vi "RotationApplication V4.vi"() -> ()   [LabVIEW 2012]
uses:
  <instrlib>/ZaberTSeries/Public/Utility/Request.ctl
  <instrlib>/ZaberTSeries/Public/Utility/Response.ctl
  Stage Global.vi
  <instrlib>/ZaberTSeries/ZaberTSeries.lvlib
panel:
  out "Scanning?":bool
  out "Current Angle (deg)":dbl=45.0
  out "Stage Position (mm)":dbl=75.00015258789062
  in  "Time Step (ms)":dbl
  in  "Rotation f(x) (mm -> deg)":string="2.7355608145532777*x*x*x*x*x*x - 1187.125773554726*x*x*x*x*x + 214643.38075449364*x*x*x*x - 20697537.088212848*x*x*x + 1122597496.9922702*x*x - 32472066742.439888*x + 391350879609.55573"
  in  "Finish Rotation f(x)":bool
  in  "Scan":bool
  in  "stop":bool
  in  "Go Home":bool
  in  "Set Home Offset":dbl=89.0
  in  "?":T1(tab)
  in  "Optimize":bool
  in  "Angle?":bool
  out "Current Angle (deg)":dbl=38.0090625
  in  "Move Rel?":bool
  in  "Move Abs?":bool
  in  "Move Rel (deg)":dbl=-1.0 step=0.1
  in  "Move Abs (deg)":dbl=19.0
  in  "Send":bool
  out "Command?":bool
  in  "REQUEST:":T2={"Device Number"=1, "Command"=23, "Data"=-10000, "Response Count"=1} {"Command" items=["Echo"=55, "Home"=1, "Move Absolute"=20, "Move Relative"=21, "Move at Constant Speed"=22, "Renumber"=2, "Restore Settings"=36, "Stop"=23]}
  out "Response Data:":T3 {"Command" items=["Constant Speed Tracking"=8, "Echo"=55, "Error"=255, "Home"=1, "Limit Active"=9, "Manual Move Tracking"=10, "Move Absolute"=20, "Move at Constant Speed"=22, "Move Relative"=21, "Renumber"=2, "Restore Settings"=36, "Stop"=23]}
  in  "Command":bool
  in  "DONE":bool=TRUE
  in  "Simulation":bool
  out "Simulate?":bool
  in  "Finish Stage":bool
  in  "Start/pause":bool
  in  "Start/Pause Stage":bool
  out "Current Position (mm)":dbl
  in  "Finish Rotation":bool
  out "Current Angle":dbl
  in  "Initial Position (mm)":dbl
  in  "Final Position (mm)":dbl
  in  "Number of Steps":u32
  in  "Speed (um/s)":dbl
  in  "Final Angle (deg)":dbl=45.0
  in  "Number of Rotations":u32=4500
  in  "Polynomial Degree":dbl=1.0
  in  "VISA reference name:":refnum<visa-resource-name>="COM4"
  # "==>"
  # "Device"
  # "Command (Binary)"
  # "Data"
  # "==>"
  # "Data"
  # "==>"
  # "Rotation Mount Settings:"
  # "Simulated Delay Stage Settings:"
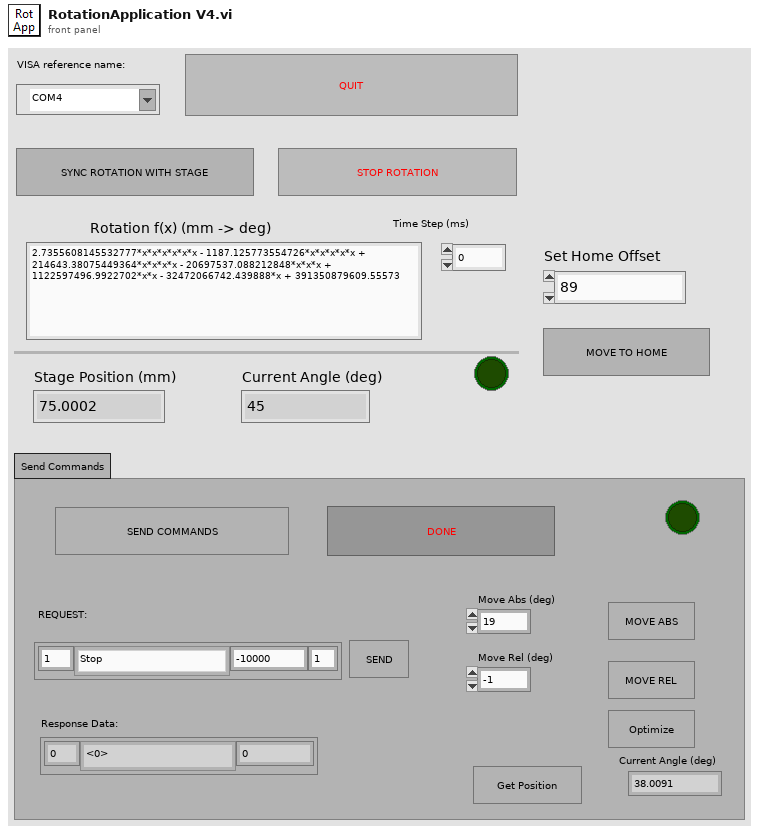
[diagram p1: front panel]
types:
  T1 = enum32{"Send Commands", "Simulated f(x)  ", "Adjust Simulation Settings"}
  T2 = typedef "ZaberTSeries.lvlib/Request.ctl" = cluster{"Device Number":u8, "Command":u8, "Data":i32, "Response Count":i32}
  T3 = typedef "ZaberTSeries.lvlib/Response.ctl" = cluster{"Device Number":u8, "Command":u8, "Data":i32}
  T4 = enum8{"Enabled", "Disabled", "Disabled and Grayed Out"}
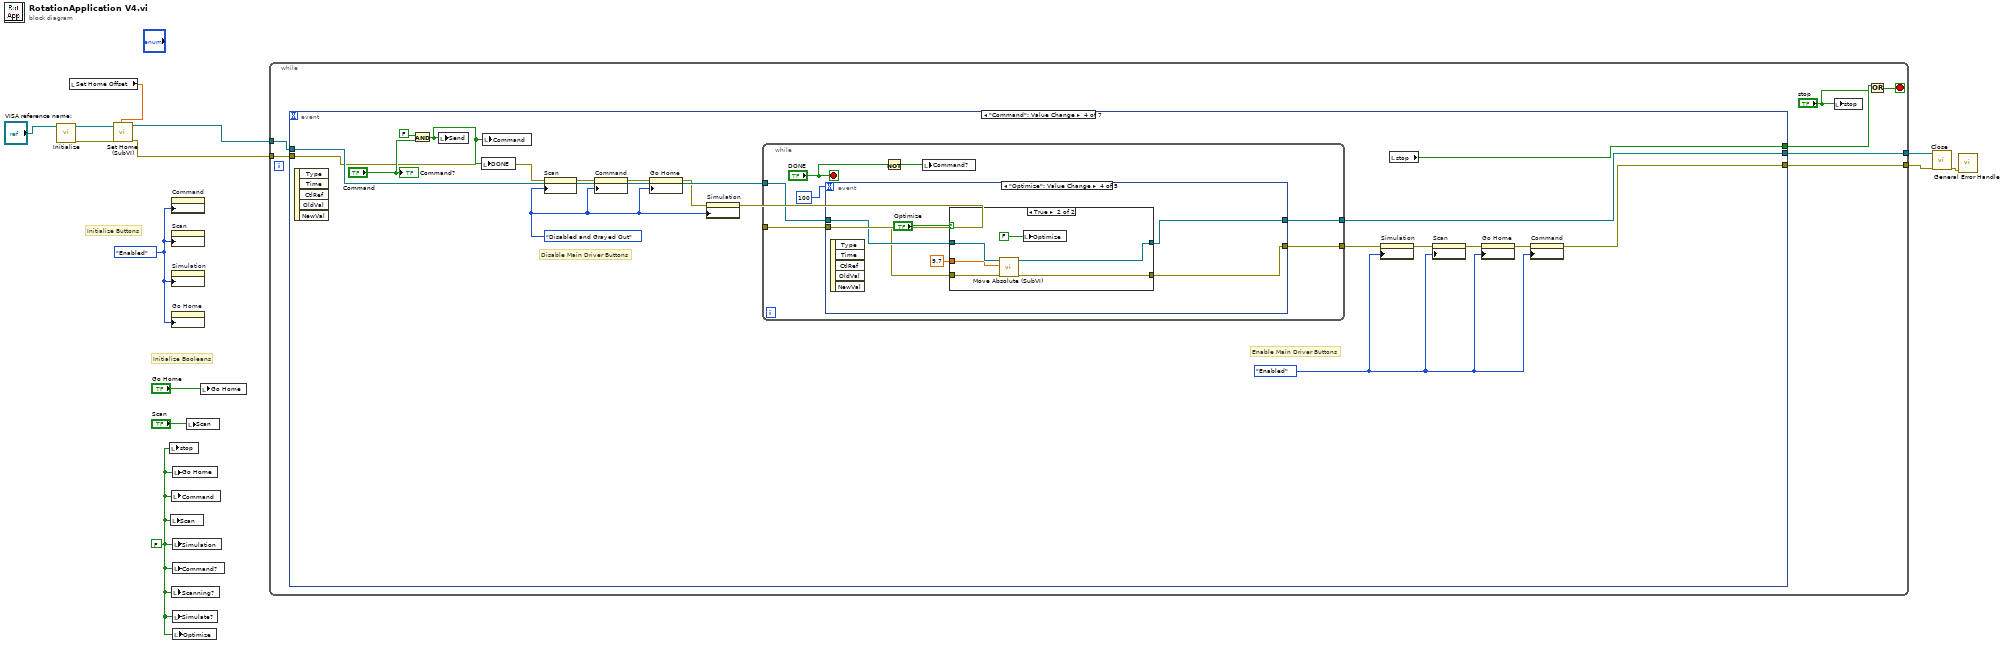
[diagram p0: block diagram]
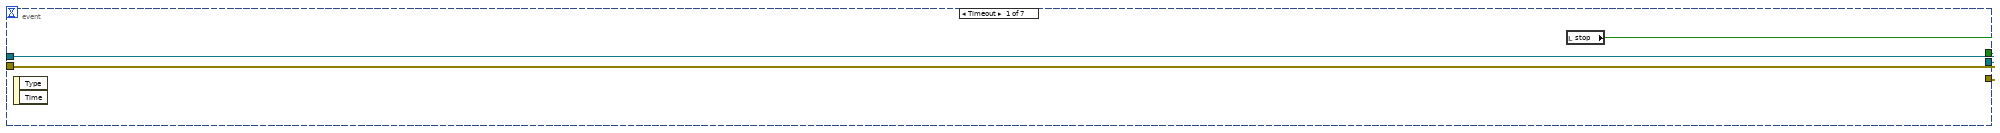
[diagram p2: hidden frame]
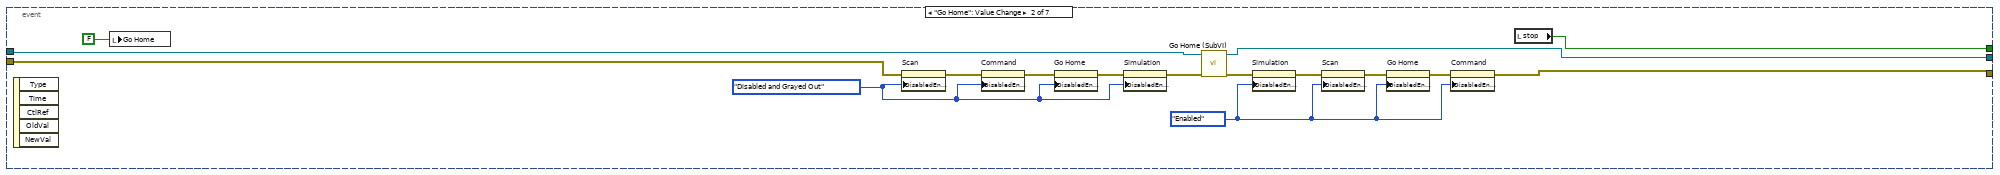
[diagram p3: hidden frame]
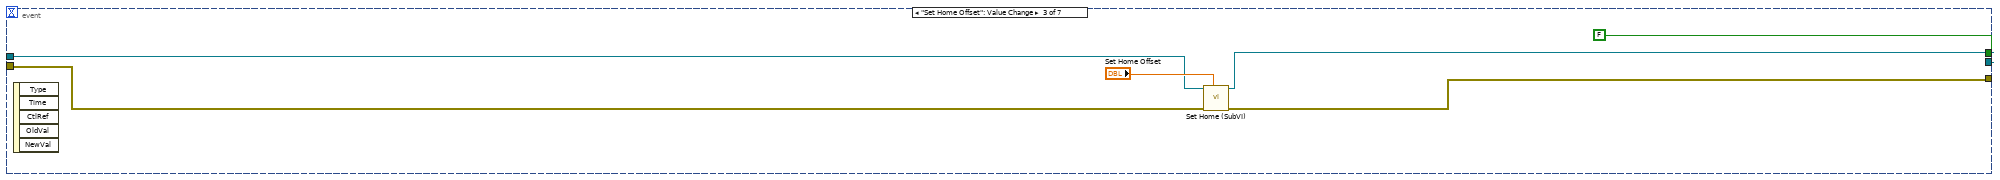
[diagram p4: hidden frame]
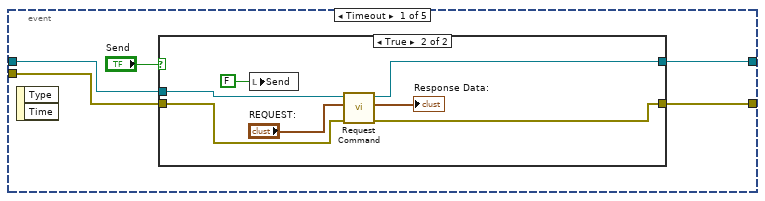
[diagram p5: hidden frame]
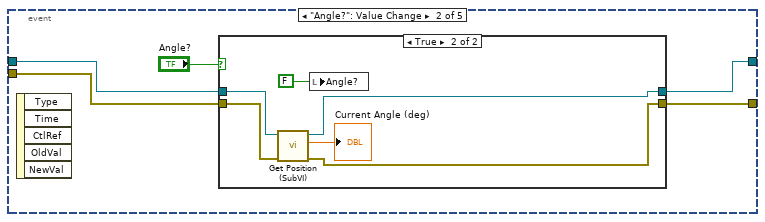
[diagram p7: hidden frame]
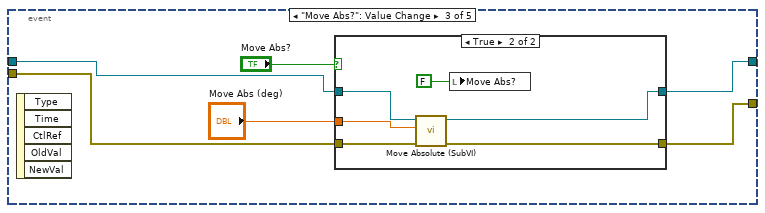
[diagram p9: hidden frame]
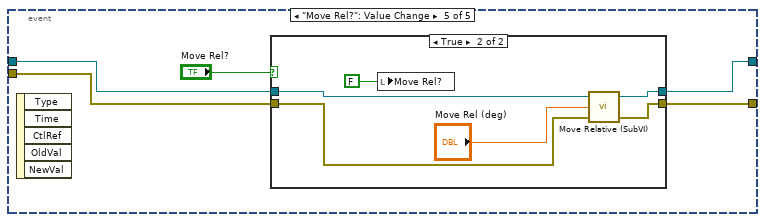
[diagram p12: hidden frame]
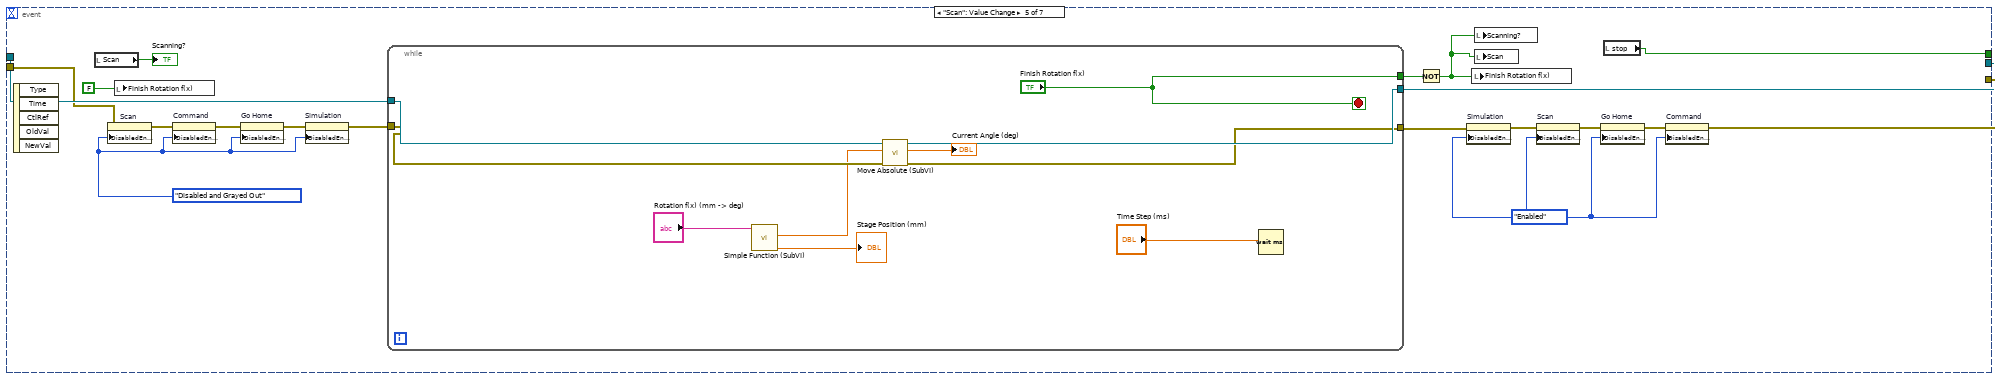
[diagram p14: hidden frame]
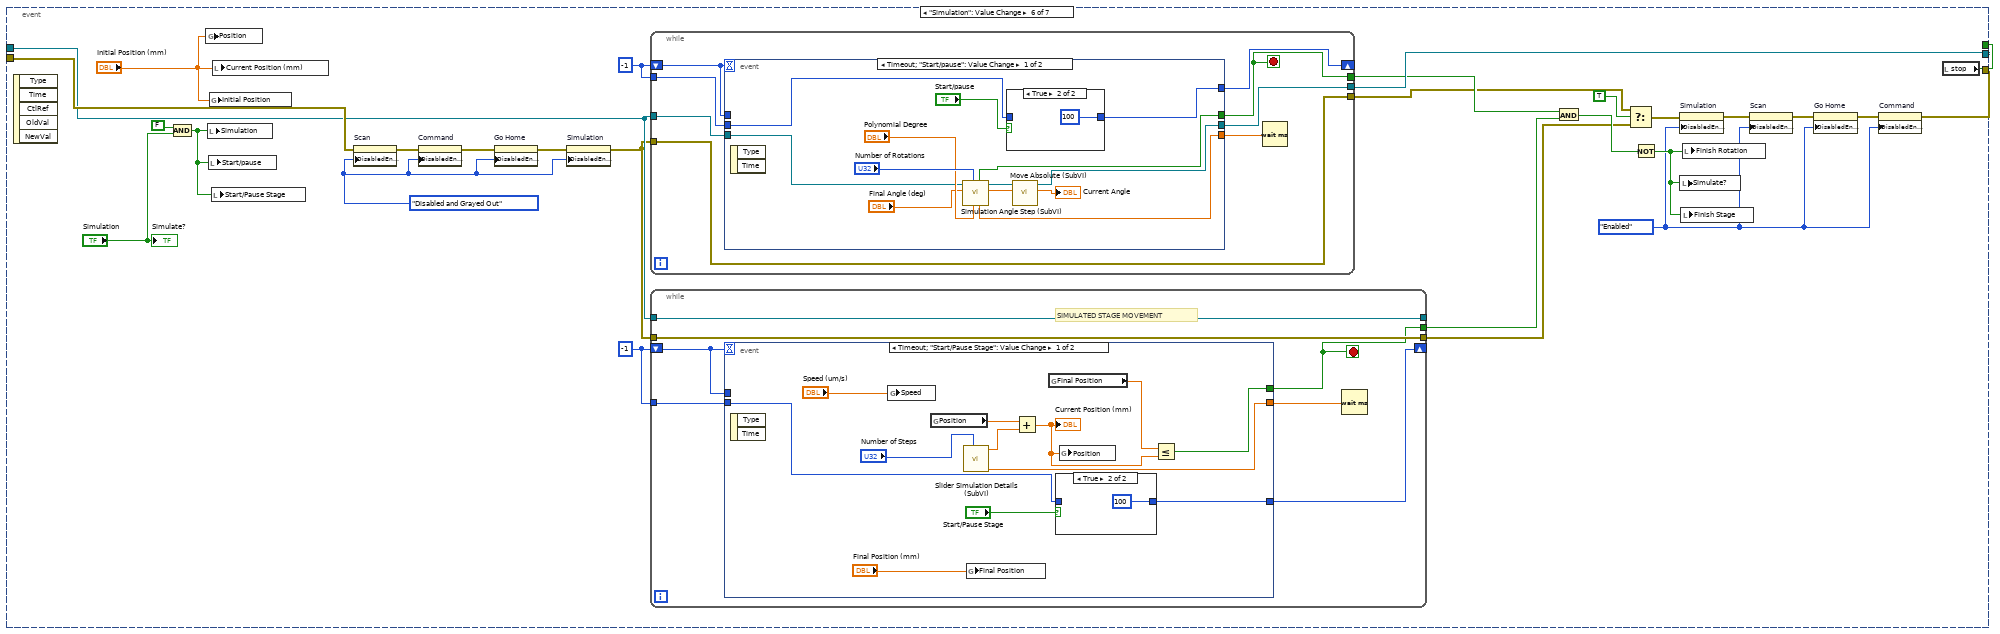
[diagram p15: hidden frame]
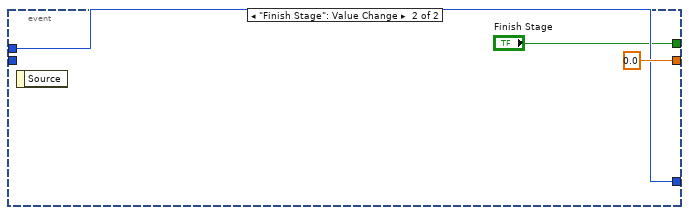
[diagram p17: hidden frame]
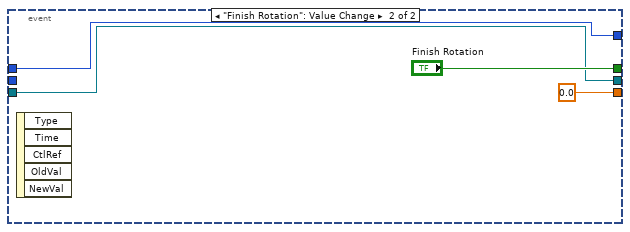
[diagram p19: hidden frame]
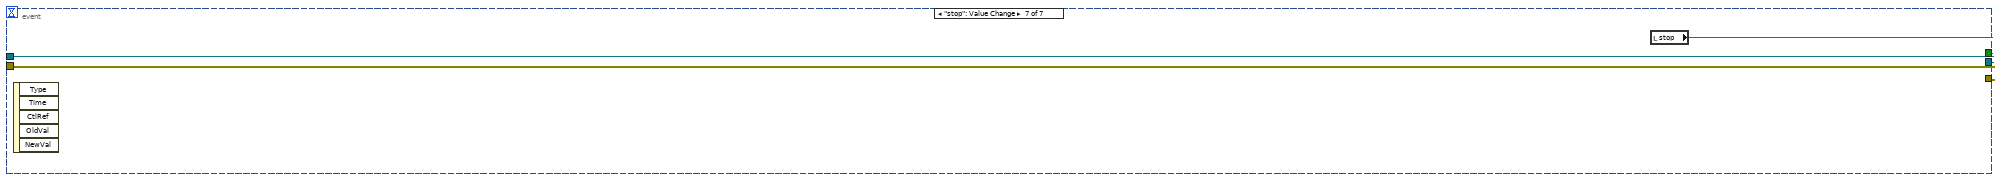
[diagram p20: hidden frame]
diagram:
  w9 = T4."Enabled" ("Disabled")
  w1 = FALSE ("y")
  # "Initialize Buttons"
  # "Initialize Booleans"
  n1 = call <instrlib>:"Initialize.vi"("VISA resource name"="VISA reference name:") -> ("error out"=w4:errorcluster, "VISA resource name out"=w6:refnum<visa-resource-name>)  [unwired: 8 in, 1 out]
  n2 = local read "Set Home Offset"() -> (w2:dbl)
  n3 = call "Set Home (SubVI).vi"("Home Offset (deg)"=w2, "error in (no error)"=w4, "VISA Refnum in"=w6) -> ("error out"=w3:errorcluster, "VISA Refnum out"=w5:refnum<visa-resource-name>)  [unwired: 7 in]
  n4 = local write "stop"(w1) -> ()
  n5 = local write "Scan"(w1) -> ()
  n6 = property on="Command" class="Bool (strict)"("DisabledEnum"=w9) -> ()  [unwired: 2 in, 2 out]
  n7 = property on="Scan" class="Bool (strict)"("DisabledEnum"=w9) -> ()  [unwired: 2 in, 2 out]
  n8 = property on="Simulation" class="Bool (strict)"("DisabledEnum"=w9) -> ()  [unwired: 2 in, 2 out]
  n9 = property on="Go Home" class="Bool (strict)"("DisabledEnum"=w9) -> ()  [unwired: 2 in, 2 out]
  n10 = local write "Command"(w1) -> ()
  n11 = local write "Scanning?"(w1) -> ()
  n12 = local write "Go Home"(w1) -> ()
  n13 = local write "Simulation"(w1) -> ()
  n14 = local write "Command?"(w1) -> ()
  n15 = local write "Simulate?"(w1) -> ()
  n16 = local write "Optimize"(w1) -> ()
  n17 = local write "Scan"("Scan") -> ()
  n18 = local write "Go Home"("Go Home") -> ()
  n19 = while {
    tunnel: w5 -> [w15]
    tunnel: w3 -> [w14]
    tunnel: [w20] -> w11
    tunnel: [w19] -> w13
    stop <- w18 stop-if-true
    n20 = event shown="[3] \"Command\": Value Change" {
      selector: _ -> [_ _ _ _ _ _ _]
      dyn-events: _ -> [_ _ _ _ _ _ _]
      timeout: _ -> [_ _ _ _ _ _ _]
      tunnel: w15 -> [w23 w34 w44 w63 w156 w183 w248]
      tunnel: w14 -> [w22 w25 w43 w47 w153 w192 w247]
      tunnel: [w23 w28 w42 w55 w155 w190 w248] -> w19
      tunnel: [w22 w29 w41 w51 w150 w187 w247] -> w20
      tunnel: [w21 w39 FALSE ("stop") w62 w157 w195 w249] -> w17
      event Timeout {
        n21 = event-data() -> ()  [unwired: 1 in, 2 out]
        n22 = local read "stop"() -> (w21:bool)
      }
      event "Go Home": Value Change {
        w26 = T4."Enabled" ("Disabled")
        w27 = T4."Disabled and Grayed Out" ("Disabled")
        n23 = event-data() -> ()  [unwired: 1 in, 5 out]
        n24 = local write "Go Home"(FALSE ("Go Home")) -> ()
        n25 = property on="Scan" class="Bool (strict)"(error in=w25, "DisabledEnum"=w27) -> (error out=w37:errorcluster)  [unwired: 1 in, 1 out]
        n26 = property on="Command" class="Bool (strict)"(error in=w37, "DisabledEnum"=w27) -> (error out=w36:errorcluster)  [unwired: 1 in, 1 out]
        n27 = property on="Go Home" class="Bool (strict)"(error in=w36, "DisabledEnum"=w27) -> (error out=w35:errorcluster)  [unwired: 1 in, 1 out]
        n28 = property on="Simulation" class="Bool (strict)"(error in=w35, "DisabledEnum"=w27) -> (error out=w33:errorcluster)  [unwired: 1 in, 1 out]
        n29 = call "Go Home (SubVI).vi"("error in (no error)"=w33, "VISA Refnum in"=w34) -> ("error out"=w24:errorcluster, "VISA Refnum out"=w28:refnum<visa-resource-name>)  [unwired: 8 in]
        n30 = property on="Simulation" class="Bool (strict)"(error in=w24, "DisabledEnum"=w26) -> (error out=w30:errorcluster)  [unwired: 1 in, 1 out]
        n31 = property on="Scan" class="Bool (strict)"(error in=w30, "DisabledEnum"=w26) -> (error out=w32:errorcluster)  [unwired: 1 in, 1 out]
        n32 = property on="Go Home" class="Bool (strict)"(error in=w32, "DisabledEnum"=w26) -> (error out=w31:errorcluster)  [unwired: 1 in, 1 out]
        n33 = property on="Command" class="Bool (strict)"(error in=w31, "DisabledEnum"=w26) -> (error out=w29:errorcluster)  [unwired: 1 in, 1 out]
        n34 = local read "stop"() -> (w39:bool)
      }
      event "Set Home Offset": Value Change {
        n35 = event-data() -> ()  [unwired: 1 in, 5 out]
        n36 = call "Set Home (SubVI).vi"("Home Offset (deg)"="Set Home Offset", "error in (no error)"=w43, "VISA Refnum in"=w44) -> ("error out"=w41:errorcluster, "VISA Refnum out"=w42:refnum<visa-resource-name>)  [unwired: 7 in]
      }
      event "Command": Value Change {
        w49 = T4."Enabled" ("Disabled")
        w50 = T4."Disabled and Grayed Out" ("Disabled")
        # "Enable Main Driver Buttons"
        # "Disable Main Driver Buttons"
        n37 = event-data() -> ()  [unwired: 1 in, 5 out]
        n38 = And(x=FALSE ("Command"), y="Command") -> (x .and. y?=w48:bool)
        n39 = local write "Send"(w48) -> ()
        n40 = local write "DONE"(w48) -> ()
        n41 = local write "Command"(w48) -> ()
        n42 = property on="Scan" class="Bool (strict)"(error in=w47, "DisabledEnum"=w50) -> (error out=w57:errorcluster)  [unwired: 1 in, 1 out]
        n43 = property on="Command" class="Bool (strict)"(error in=w57, "DisabledEnum"=w50) -> (error out=w58:errorcluster)  [unwired: 1 in, 1 out]
        n44 = property on="Go Home" class="Bool (strict)"(error in=w58, "DisabledEnum"=w50) -> (error out=w59:errorcluster)  [unwired: 1 in, 1 out]
        n45 = property on="Simulation" class="Bool (strict)"(error in=w59, "DisabledEnum"=w50) -> (error out=w56:errorcluster)  [unwired: 1 in, 1 out]
        n46 = while {
          tunnel: w63 -> [w66]
          tunnel: [w70] -> w55
          tunnel: w56 -> [w65]
          tunnel: [w69] -> w46
          stop <- "DONE" stop-if-true
          n47 = event shown="[3] \"Optimize\": Value Change" {
            selector: _ -> [_ _ _ _ _]
            dyn-events: _ -> [_ _ _ _ _]
            timeout: 100 -> [_ _ _ _ _]
            tunnel: [w75 w88 w100 w113 w127] -> w70
            tunnel: [w74 w85 w98 w112 w126] -> w69
            tunnel: w66 -> [w72 w87 w101 w116 w129]
            tunnel: w65 -> [w71 w86 w99 w114 w128]
            event Timeout {
              n48 = event-data() -> ()  [unwired: 1 in, 2 out]
              n49 = case shown="True" "Send" {
                tunnel: w72 -> [w77 w83]
                tunnel: [w77 w82] -> w75
                tunnel: w71 -> [w76 w81]
                tunnel: [w76 w80] -> w74
                frame False {
                }
                frame True {
                  n50 = local write "Send"(FALSE ("Send")) -> ()
                  n51 = call <instrlib>:"Request Command.vi"("error in (no error)"=w81, "Request"="REQUEST:", "VISA resource name"=w83) -> ("error out"=w80:errorcluster, "First Response"=→"Response Data:":T3, "VISA resource name out"=w82:refnum<visa-resource-name>)  [unwired: 5 in, 1 out]
                }
              }
            }
            event "Angle?": Value Change {
              n52 = event-data() -> ()  [unwired: 1 in, 5 out]
              n53 = case shown="True" "Angle?" {
                tunnel: [w91 w96] -> w88
                tunnel: w87 -> [w91 w95]
                tunnel: w86 -> [w90 w94]
                tunnel: [w90 w93] -> w85
                frame False {
                }
                frame True {
                  n54 = call "Get Position (SubVI).vi"("error in (no error)"=w94, "VISA Refnum in"=w95) -> ("error out"=w93:errorcluster, "Position"=→"Current Angle (deg)":dbl, "VISA Refnum out"=w96:refnum<visa-resource-name>)  [unwired: 7 in]
                  n55 = local write "Angle?"(FALSE ("Angle?")) -> ()
                }
              }
            }
            event "Move Abs?": Value Change {
              n56 = event-data() -> ()  [unwired: 1 in, 5 out]
              n57 = case shown="True" "Move Abs?" {
                tunnel: "Move Abs (deg)" -> [_ w107]
                tunnel: w101 -> [w105 w111]
                tunnel: [w105 w110] -> w100
                tunnel: w99 -> [w104 w109]
                tunnel: [w104 w108] -> w98
                frame False {
                }
                frame True {
                  n58 = call "Move Absolute (SubVI).vi"("error in (no error)"=w109, "Move to Angle"=w107, "VISA Refnum in"=w111) -> ("error out"=w108:errorcluster, "VISA Refnum out"=w110:refnum<visa-resource-name>)  [unwired: 6 in, 1 out]
                  n59 = local write "Move Abs?"(FALSE ("Move Abs?")) -> ()
                }
              }
            }
            event "Optimize": Value Change {
              n60 = event-data() -> ()  [unwired: 1 in, 5 out]
              n61 = case shown="True" "Optimize" {
                tunnel: 9.7 ("Move Abs (deg)") -> [_ w121]
                tunnel: w116 -> [w119 w125]
                tunnel: [w119 w124] -> w113
                tunnel: w114 -> [w118 w123]
                tunnel: [w118 w122] -> w112
                frame False {
                }
                frame True {
                  n62 = call "Move Absolute (SubVI).vi"("error in (no error)"=w123, "Move to Angle"=w121, "VISA Refnum in"=w125) -> ("error out"=w122:errorcluster, "VISA Refnum out"=w124:refnum<visa-resource-name>)  [unwired: 6 in, 1 out]
                  n63 = local write "Optimize"(FALSE ("Move Abs?")) -> ()
                }
              }
            }
            event "Move Rel?": Value Change {
              n64 = event-data() -> ()  [unwired: 1 in, 5 out]
              n65 = case shown="True" "Move Rel?" {
                tunnel: w129 -> [w132 w137]
                tunnel: w128 -> [w131 w136]
                tunnel: [w132 w134] -> w127
                tunnel: [w131 w135] -> w126
                frame False {
                }
                frame True {
                  n66 = local write "Move Rel?"(FALSE ("Move Rel?")) -> ()
                  n67 = call "Move Relative (SubVI).vi"("error in (no error)"=w136, "Degrees to move"="Move Rel (deg)", "VISA resource name"=w137) -> ("error out"=w135:errorcluster, "VISA resource name out"=w134:refnum<visa-resource-name>)  [unwired: 1 out]
                }
              }
            }
          }
          n68 = Not(x="DONE") -> (.not. x?=w67:bool)
          n69 = local write "Command?"(w67) -> ()
        }
        n70 = property on="Simulation" class="Bool (strict)"(error in=w46, "DisabledEnum"=w49) -> (error out=w52:errorcluster)  [unwired: 1 in, 1 out]
        n71 = local read "stop"() -> (w62:bool)
        n72 = property on="Scan" class="Bool (strict)"(error in=w52, "DisabledEnum"=w49) -> (error out=w54:errorcluster)  [unwired: 1 in, 1 out]
        n73 = property on="Go Home" class="Bool (strict)"(error in=w54, "DisabledEnum"=w49) -> (error out=w53:errorcluster)  [unwired: 1 in, 1 out]
        n74 = property on="Command" class="Bool (strict)"(error in=w53, "DisabledEnum"=w49) -> (error out=w51:errorcluster)  [unwired: 1 in, 1 out]
        "Command?" <- "Command"
      }
      event "Scan": Value Change {
        w143 = T4."Enabled" ("Disabled")
        w144 = T4."Disabled and Grayed Out" ("Disabled")
        n75 = event-data() -> ()  [unwired: 1 in, 5 out]
        n76 = local read "Scan"() -> (→"Scanning?":bool)
        n77 = property on="Scan" class="Bool (strict)"(error in=w153, "DisabledEnum"=w144) -> (error out=w152:errorcluster)  [unwired: 1 in, 1 out]
        n78 = local write "Finish Rotation f(x)"(FALSE ("Command")) -> ()
        n79 = property on="Command" class="Bool (strict)"(error in=w152, "DisabledEnum"=w144) -> (error out=w154:errorcluster)  [unwired: 1 in, 1 out]
        n80 = property on="Go Home" class="Bool (strict)"(error in=w154, "DisabledEnum"=w144) -> (error out=w147:errorcluster)  [unwired: 1 in, 1 out]
        n81 = property on="Simulation" class="Bool (strict)"(error in=w147, "DisabledEnum"=w144) -> (error out=w148:errorcluster)  [unwired: 1 in, 1 out]
        n82 = while {
          tunnel: w156 -> [w167]
          tunnel: [w166] -> w155
          tunnel: w148 -> [w165]
          tunnel: [w164] -> w145
          tunnel: ["Finish Rotation f(x)"] -> w139
          stop <- "Finish Rotation f(x)" stop-if-true
          n83 = call "Simple Function (SubVI).vi"("f(x) (mm -> deg)"="Rotation f(x) (mm -> deg)") -> ("Stage Position (mm)"=→"Stage Position (mm)":dbl, "Next Angle (deg)"=w161:dbl)  [unwired: 9 in]
          n84 = call "Move Absolute (SubVI).vi"("error in (no error)"=w165, "Move to Angle"=w161, "VISA Refnum in"=w167) -> ("error out"=w164:errorcluster, "New Angle"=→"Current Angle (deg)":dbl, "VISA Refnum out"=w166:refnum<visa-resource-name>)  [unwired: 6 in]
          n85 = Wait (ms)(milliseconds to wait="Time Step (ms)") -> ()  [unwired: 1 out]
        }
        n86 = Not(x=w139) -> (.not. x?=w140:bool)
        n87 = property on="Simulation" class="Bool (strict)"(error in=w145, "DisabledEnum"=w143) -> (error out=w146:errorcluster)  [unwired: 1 in, 1 out]
        n88 = local write "Finish Rotation f(x)"(w140) -> ()
        n89 = local write "Scanning?"(w140) -> ()
        n90 = local write "Scan"(w140) -> ()
        n91 = property on="Scan" class="Bool (strict)"(error in=w146, "DisabledEnum"=w143) -> (error out=w149:errorcluster)  [unwired: 1 in, 1 out]
        n92 = property on="Go Home" class="Bool (strict)"(error in=w149, "DisabledEnum"=w143) -> (error out=w151:errorcluster)  [unwired: 1 in, 1 out]
        n93 = local read "stop"() -> (w157:bool)
        n94 = property on="Command" class="Bool (strict)"(error in=w151, "DisabledEnum"=w143) -> (error out=w150:errorcluster)  [unwired: 1 in, 1 out]
      }
      event "Simulation": Value Change {
        w177 = -1
        w176 = -1
        w168 = T4."Enabled" ("Disabled")
        w169 = T4."Disabled and Grayed Out" ("Disabled")
        n95 = event-data() -> ()  [unwired: 1 in, 5 out]
        n96 = And(x=FALSE ("Command"), y="Simulation") -> (x .and. y?=w170:bool)
        n97 = global write "Stage Global.vi" "Position"("Initial Position (mm)") -> ()
        n98 = local write "Simulation"(w170) -> ()
        n99 = local write "Start/pause"(w170) -> ()
        n100 = global write "Stage Global.vi" "Initial Position"("Initial Position (mm)") -> ()
        n101 = local write "Start/Pause Stage"(w170) -> ()
        n102 = local write "Current Position (mm)"("Initial Position (mm)") -> ()
        n103 = property on="Scan" class="Bool (strict)"(error in=w192, "DisabledEnum"=w169) -> (error out=w194:errorcluster)  [unwired: 1 in, 1 out]
        n104 = property on="Command" class="Bool (strict)"(error in=w194, "DisabledEnum"=w169) -> (error out=w193:errorcluster)  [unwired: 1 in, 1 out]
        n105 = property on="Go Home" class="Bool (strict)"(error in=w193, "DisabledEnum"=w169) -> (error out=w191:errorcluster)  [unwired: 1 in, 1 out]
        n106 = property on="Simulation" class="Bool (strict)"(error in=w191, "DisabledEnum"=w169) -> (error out=w182:errorcluster)  [unwired: 1 in, 1 out]
        n107 = while {
          tunnel: w182 -> [w227]
          tunnel: w183 -> [w222]
          tunnel: [w221] -> w190
          tunnel: [w227] -> w173
          tunnel: [w226] -> w179
          shift-right: [w225] -> _
          shift-left: w177 -> [w223]
          tunnel: w177 -> [w224]
          stop <- w226 stop-if-true
          n108 = event shown="[0] Timeout;  \"Start/pause\": Value Change" {
            selector: _ -> [_ _]
            dyn-events: _ -> [_ _]
            timeout: w223 -> [_ _]
            tunnel: [w228 "Finish Rotation"] -> w226
            tunnel: [w239 w245] -> w225
            tunnel: w224 -> [w238 _]
            tunnel: w223 -> [_ w245]
            tunnel: w222 -> [w233 w244]
            tunnel: [w232 w244] -> w221
            tunnel: [w231 0.0 ("Angle Time Step (ms)")] -> w220
            event Timeout; "Start/pause": Value Change {
              n109 = event-data() -> ()  [unwired: 1 in, 2 out]
              n110 = call "Simulation Angle Step (SubVI).vi"("n"="Polynomial Degree", "N (Rot)"="Number of Rotations", "Final Angle"="Final Angle (deg)", "VISA Refnum in"=w233) -> ("Next Angle"=w235:dbl, "VISA Refnum out"=w234:refnum<visa-resource-name>, "Angle Time Step (ms)"=w231:dbl, "Rotation Complete?"=w228:bool)  [unwired: 3 in, 1 out]
              n111 = case shown="True" "Start/pause" {
                tunnel: [w241 100] -> w239
                tunnel: w238 -> [w241 _]
                frame False {
                }
                frame True {
                }
              }
              n112 = call "Move Absolute (SubVI).vi"("Move to Angle"=w235, "VISA Refnum in"=w234) -> ("New Angle"=→"Current Angle":dbl, "VISA Refnum out"=w232:refnum<visa-resource-name>)  [unwired: 7 in, 1 out]
            }
            event "Finish Rotation": Value Change {
              n113 = event-data() -> ()  [unwired: 1 in, 5 out]
            }
          }
          n114 = Wait (ms)(milliseconds to wait=w220) -> ()  [unwired: 1 out]
        }
        n115 = while {
          tunnel: w182 -> [w201]
          tunnel: w183 -> [w202]
          tunnel: [w202] -> _
          tunnel: [w201] -> w174
          shift-right: [w198] -> _
          shift-left: w176 -> [w199]
          tunnel: [w197] -> w178
          tunnel: w176 -> [w196]
          stop <- w197 stop-if-true
          # "SIMULATED STAGE MOVEMENT"
          n116 = event shown="[0] Timeout;  \"Start/Pause Stage\": Value Change" {
            selector: _ -> [_ _]
            dyn-events: _ -> [_ _]
            timeout: w199 -> [_ _]
            tunnel: [w212 "Finish Stage"] -> w197
            tunnel: [w214 w218] -> w198
            tunnel: w199 -> [_ w218]
            tunnel: [w213 0.0 ("Time Between Steps (ms)")] -> w200
            tunnel: w196 -> [w206 _]
            event Timeout; "Start/Pause Stage": Value Change {
              n117 = event-data() -> ()  [unwired: 1 in, 2 out]
              n118 = global write "Stage Global.vi" "Speed"("Speed (um/s)") -> ()
              n119 = global read "Stage Global.vi" "Position"() -> (w208:dbl)
              n120 = call "Slider Simulation Details (SubVI).vi"("Number of Steps"="Number of Steps") -> ("Time Between Steps (ms)"=w213:dbl, "Step Size (mm)"=w204:dbl)  [unwired: 9 in]
              n121 = global write "Stage Global.vi" "Final Position"("Final Position (mm)") -> ()
              n122 = Add(x=w208, y=w204) -> (x+y=w203:dbl)
              "Current Position (mm)" <- w203
              n123 = global read "Stage Global.vi" "Final Position"() -> (w205:dbl)
              n124 = case shown="True" "Start/Pause Stage" {
                tunnel: [w215 100] -> w214
                tunnel: w206 -> [w215 _]
                frame False {
                }
                frame True {
                }
              }
              n125 = global write "Stage Global.vi" "Position"(w203) -> ()
              n126 = Less Or Equal?(x=w205, y=w203) -> (x <= y?=w212:bool)
            }
            event "Finish Stage": Value Change {
              n127 = event-data() -> ()  [unwired: 1 in, 1 out]
            }
          }
          n128 = Wait (ms)(milliseconds to wait=w200) -> ()  [unwired: 1 out]
        }
        n129 = And(x=w179, y=w178) -> (x .and. y?=w180:bool)
        n130 = Select(t=w173, s=TRUE, f=w174) -> (s? t:f=w172:errorcluster)
        n131 = Not(x=w180) -> (.not. x?=w171:bool)
        n132 = property on="Simulation" class="Bool (strict)"(error in=w172, "DisabledEnum"=w168) -> (error out=w186:errorcluster)  [unwired: 1 in, 1 out]
        n133 = local write "Simulate?"(w171) -> ()
        n134 = local write "Finish Stage"(w171) -> ()
        n135 = local write "Finish Rotation"(w171) -> ()
        n136 = property on="Scan" class="Bool (strict)"(error in=w186, "DisabledEnum"=w168) -> (error out=w189:errorcluster)  [unwired: 1 in, 1 out]
        n137 = property on="Go Home" class="Bool (strict)"(error in=w189, "DisabledEnum"=w168) -> (error out=w188:errorcluster)  [unwired: 1 in, 1 out]
        n138 = property on="Command" class="Bool (strict)"(error in=w188, "DisabledEnum"=w168) -> (error out=w187:errorcluster)  [unwired: 1 in, 1 out]
        n139 = local read "stop"() -> (w195:bool)
        "Simulate?" <- "Simulation"
      }
      event "stop": Value Change {
        n140 = event-data() -> ()  [unwired: 1 in, 5 out]
        n141 = local read "stop"() -> (w249:bool)
      }
    }
    n142 = local write "stop"("stop") -> ()
    n143 = Or(x=w17, y="stop") -> (x .or. y?=w18:bool)
  }
  n144 = call <instrlib>:"Close.vi"("error in (no error)"=w11, "VISA resource name"=w13) -> ("error out"=w10:errorcluster)  [unwired: 8 in, 1 out]
  n145 = call <vilib>:"General Error Handler.vi"("error in (no error)"=w10) -> ()  [unwired: 10 in, 5 out]
